vi "xbox.vi"() -> ()   [LabVIEW 2017]
panel:
  in  "STOP":bool
  # "XBOX controller reader"
  # "This program acts as a server\nand shares the output of the\nXBOX controller to other\ncomputers via the network.\nYou can (re)start and stop it\nindependently."
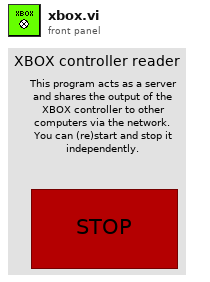
[diagram p1: front panel]
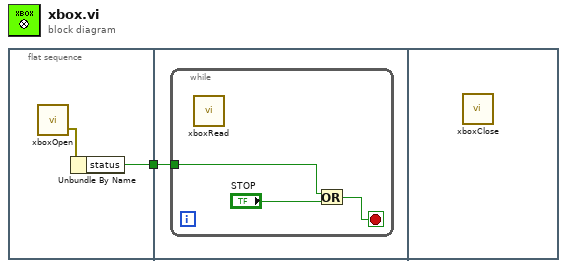
[diagram p0: block diagram]
diagram:
  n1 = flat-sequence {
    tunnel: [w2] -> w1
    tunnel: w1 -> [w4]
    frame #0 {
      n2 = call "xboxOpen.vi"() -> ("xboxError"=w3:errorcluster)  [unwired: 1 in, 1 out]
      n3 = Unbundle By Name(w3) -> ("status"=w2:bool)
    }
    frame #1 {
      n4 = while {
        tunnel: w4 -> [w5]
        stop <- w7 stop-if-true
        n5 = call "xboxRead.vi"() -> ()  [unwired: 2 out]
        n6 = Or(x=w5, y="STOP") -> (x .or. y?=w7:bool)
      }
    }
    frame #2 {
      n7 = call "xboxClose.vi"() -> ()  [unwired: 1 out]
    }
  }
